vi "setGrating.vi"(8 "error in (no error)":errorcluster, 9 "Monochromator in":refnum<class "Monochromator.lvclass">, 10 "GratingType":T1=enum."Red", 11 "ReadySate in":refnum<class "ReadySate.lvclass">) -> (0 "error out":errorcluster, 1 "Monochromator out":refnum<class "Monochromator.lvclass">, 3 "ReadySate out":refnum<class "ReadySate.lvclass">)   [LabVIEW 2020, in "ReadySate.lvclass"]
uses:
  ReadySate.lvclass
  Typedefs/GratingType.ctl
  Monochromator/Monochromator.lvclass
  Typedefs/SWStatus.ctl
  Typedefs/AckType.ctl
  Commands/CommandFactory/commandList.ctl
  Commands/CommandFactory/CommandFactory.lvclass
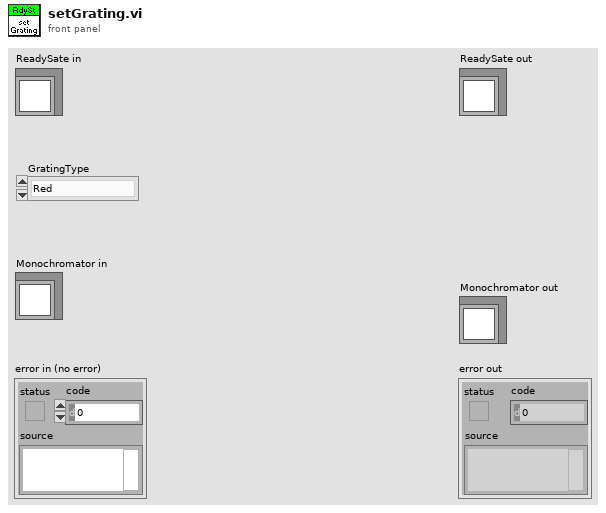
[diagram p1: front panel]
types:
  T1 = typedef "GratingType.ctl" = enum16{"Blue", "Red", "Mirror"}
  T2 = typedef "commandList.ctl" = enum16{"ChangeSlitWidth", "ChangeWavelendth", "SelectGrating"}
  T3 = typedef "AckType.ctl" = enum16{"OK", "OutOfRange", "Unknown", "Busy", "Rejected"}
  T4 = typedef "SWStatus.ctl" = enum16{"OfflineState", "ReadyState", "SettingUpState", "FaultState"}
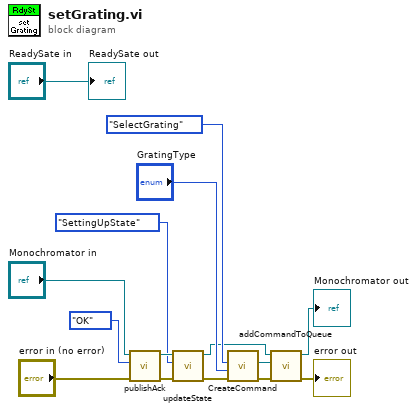
[diagram p0: block diagram]
diagram:
  n1 = call "publishAck.vi"("error in (no error)"="error in (no error)", "Ack"=AckType."OK" ("AckType"), "Monochromator in"="Monochromator in") -> ("error out"=w13:errorcluster, "Monochromator out"=w14:refnum<class "Monochromator.lvclass">)  [unwired: 7 in]
  n2 = call "updateState.vi"("error in (no error)"=w13, "SWStatus"=SWStatus."SettingUpState", "Monochromator in"=w14) -> ("error out"=w3:errorcluster, "Monochromator out"=w4:refnum<class "Monochromator.lvclass">)  [unwired: 7 in]
  n3 = call "CreateCommand.vi"("error in (no error)"=w3, "param"="GratingType", "Command"=commandList."SelectGrating") -> ("error out"=w2:errorcluster, "Command.lvclass"=w1:refnum<class "Command.lvclass">)  [unwired: 6 in, 1 out]
  n4 = call "addCommandToQueue.vi"("error in (no error)"=w2, "Command.lvclass"=w1, "Monochromator in"=w4) -> ("error out"=→"error out":errorcluster, "Monochromator out"=→"Monochromator out":refnum<class "Monochromator.lvclass">)  [unwired: 7 in]
  "ReadySate out" <- "ReadySate in"
